vi "SVT Running RMS Level (1 Ch).vi"(6 "restart averaging (F)":bool, 8 "error in (no error)":errorcluster, 9 "integration time [s]":dbl=1.0 format="%.2f", 11 "scaled signal [EU]":waveform(dbl)={"t0"=timestamp(0 s since 1904-01-01), "dt"=1.0, "Y"=[0.0]}) -> (0 "error out":errorcluster, 1 "actual integration time [s]":dbl=nan format="%.2f", 2 "unit label":string, 3 "running RMS level [EU rms]":dbl=nan format="%.2f")   [LabVIEW 2017]
doc: "Computes the running root-mean-square (RMS) level of <B>scaled signal [EU]</B> or <B>even angle signal [EU]</B>. <B>integration time [s]</B> and <B>integration revolutions</B> specify the duration over which the RMS level is computed. You can use this polymorphic VI to compute the running RMS level for a single channel or for N channels, or for a single channel or N channels of resampled data. The data type you wire to the <B>scaled signal [EU]</B> or <B>even angle signal [EU]</B> input determines the polymorphic instance to use."
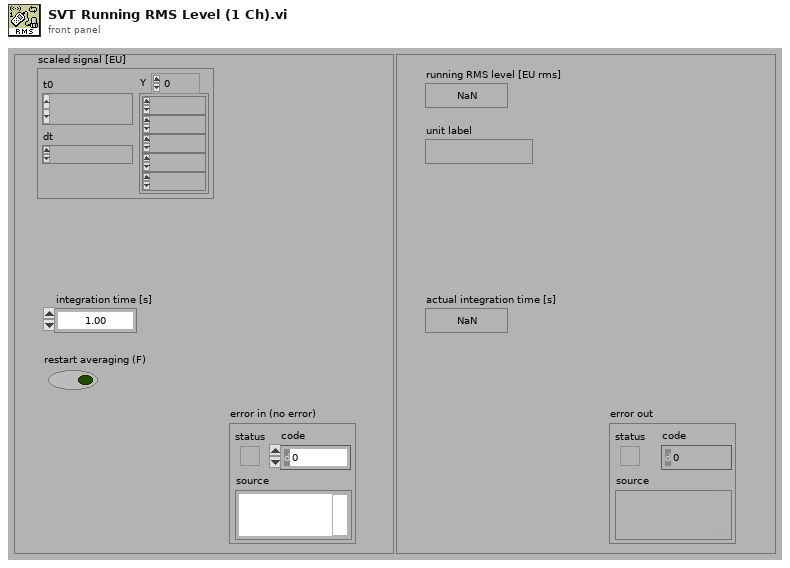
[diagram p1: front panel]
types:
  T1 = enum16{"RMS", "Running RMS", "Exp avg  ", "Dec exp avg ", "Peak", "Crest"}
  T2 = enum16{"Reset filter", "Restart averaging", "Continue processing"}
  T3 = typedef "svc_Channel Info.ctl" = cluster{"sensor sensitivity":dbl, "engineering units":T4, "dB reference":dbl, "custom label":string, "weighting filter":T5, "pregain":dbl}
  T4 = typedef "svc_Engineering Units Text Ring.ctl" = u16
  T5 = typedef "svc_Weighting Filter Text Ring.ctl" = u16
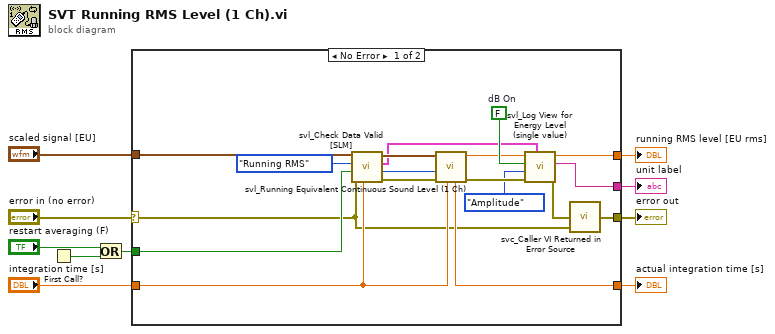
[diagram p0: block diagram]
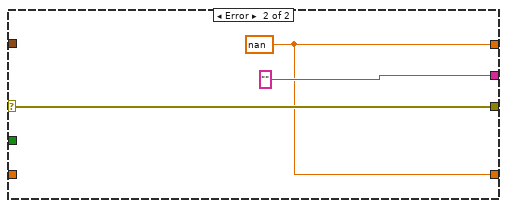
[diagram p2: hidden frame]
diagram:
  n1 = First Call?() -> (First Call?: T/F=w4:bool)
  n2 = Or(x="restart averaging (F)", y=w4) -> (x .or. y?=w3:bool)
  n3 = case shown="No Error" "error in (no error)" {
    tunnel: [w24 "" ("unit label")] -> w6
    tunnel: w3 -> [w17 _]
    tunnel: "scaled signal [EU]" -> [w14 _]
    tunnel: [w19 w29] -> w1
    selector: "error in (no error)" -> [w11 w31]
    tunnel: "integration time [s]" -> [w25 _]
    tunnel: [w26 w29] -> w9
    tunnel: [w27 w31] -> w8
    frame No Error {
      w23 = FALSE  # dB On
      n4 = call <vilib>:"svl_Check Data Valid [SLM].vi"("integration time [s]"=w25, "error in (no error)"=w11, "restart averaging (F)"=w17, "Level Analysis"=T1."Running RMS", "scaled signal [EU]"=w14) -> ("error out"=w18:errorcluster, "processing state"=w16:T2, "channel info"=w12:T3, "dup scaled signal [EU]"=w13:waveform(dbl))  [unwired: 3 in]
      n5 = call <vilib>:"svl_Running Equivalent Continuous Sound Level (1 Ch).vi"("integration time [s]"=w25, "error in (no error)"=w18, "processing state"=w16, "scaled signal"=w13) -> ("error out"=w22:errorcluster, "Running Leq"=w21:dbl, "actual integration time [s]"=w26:dbl)  [unwired: 5 in]
      n6 = call <vilib>:"svl_Log View for Energy Level (single value).vi"("channel info"=w12, "error in (no error)"=w22, "view mode"=enum16{"Power", "Amplitude"}."Amplitude", "dB On (T)"=w23, "energy level [EU^2 rms]"=w21) -> ("error out"=w28:errorcluster, "unit label"=w24:string, "energy level [EU^2 rms]"=w19:dbl)  [unwired: 4 in]
      n7 = call <vilib>:"svc_Caller VI Returned in Error Source.vi"("warning input to caller"=w11, "error in (no error)"=w28) -> ("error out"=w27:errorcluster)  [unwired: 3 in]
    }
    frame Error {
      w29 = nan ("energy level [EU^2 rms]")
    }
  }
  "running RMS level [EU rms]" <- w1
  "unit label" <- w6
  "error out" <- w8
  "actual integration time [s]" <- w9
